vi "Set Executed System Actions.vi"(8 "error in (no error)":errorcluster, 10 "Executed System Actions":string[](array[string]), 11 "TLB' Error Handler in":refnum<class "TLB` Error Handler.lvclass">) -> (0 "error out":errorcluster, 3 "TLB' Error Handler out":refnum<class "TLB` Error Handler.lvclass">)   [LabVIEW 2026, in "Synchronize AWS S3 Content.lvlib" / "TLB` Error Handler.lvclass"]
uses:
  TLB` Error Handler.lvclass
  TLB` Error Handler.lvclass/TLB` Error Handler.ctl
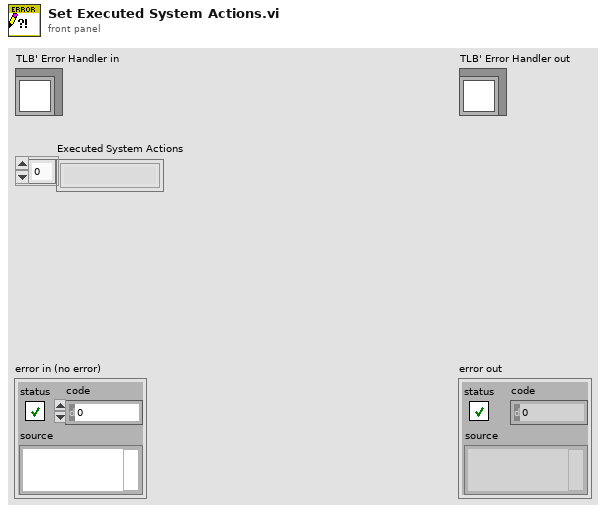
[diagram p1: front panel]
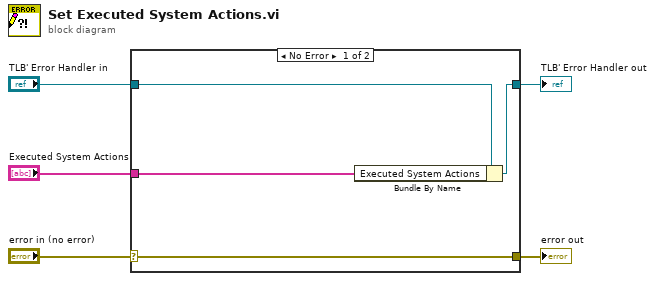
[diagram p0: block diagram]
diagram:
  n1 = case shown="No Error" "error in (no error)" {
    selector: "error in (no error)" -> [w9 w10]
    tunnel: [w9 w10] -> w4
    tunnel: [w7 w11] -> w2
    tunnel: "TLB' Error Handler in" -> [w8 w11]
    tunnel: "Executed System Actions" -> [w6 _]
    frame No Error {
      n2 = Bundle By Name(cluster=w8, "Executed System Actions"=w6) -> (w7:refnum<class "TLB` Error Handler.lvclass">)
    }
    frame Error {
    }
  }
  "error out" <- w4
  "TLB' Error Handler out" <- w2
